vi "command stage.vi"(9 "Error In":errorcluster, 11 "Command Stage":T1={"dx (um) (0 -> ignore)"=0.0, "dy (um) (0 -> ignore)"=0.0, "dz (um) (0 -> ignore)"=0.0, "Re-center x,y"=FALSE, "Re-center z"=FALSE, "x (um) (-1 -> ignore)"=-1.0, "y (um) (-1 -> ignore)"=-1.0, "z (um) (-1 -> ignore)"=-1.0}) -> (1 "Error Out":errorcluster)   [LabVIEW 2014]
uses:
  Stage Control/Stage SubVis/move stage.ctl
  Stage Control/Stage SubVis/user event out globals - SubVI.vi
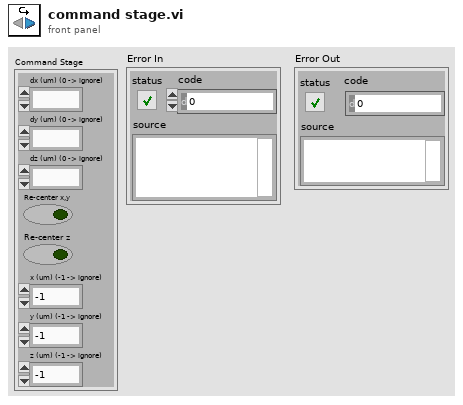
[diagram p1: front panel]
types:
  T1 = typedef "move stage.ctl" = cluster{"dx (um) (0 -> ignore)":ext, "dy (um) (0 -> ignore)":ext, "dz (um) (0 -> ignore)":ext, "Re-center x,y":bool, "Re-center z":bool, "x (um) (-1 -> ignore)":dbl, "y (um) (-1 -> ignore)":dbl, "z (um) (-1 -> ignore)":dbl}
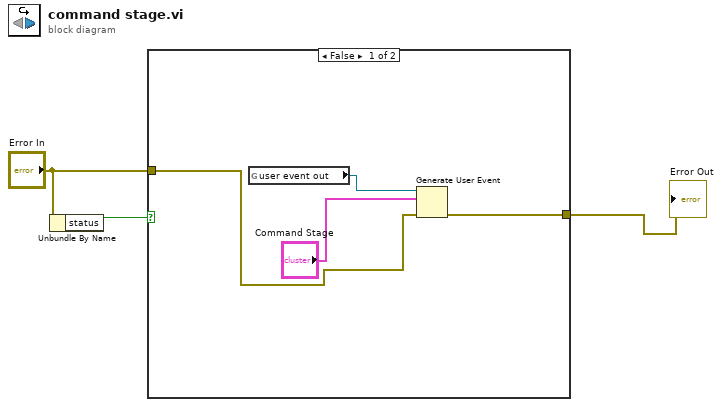
[diagram p0: block diagram]
diagram:
  n1 = Unbundle By Name("Error In") -> ("status"=w3:bool)
  n2 = case shown="False" w3 {
    tunnel: "Error In" -> [w5 w8]
    tunnel: [w4 w8] -> w1
    frame False {
      n3 = global read "user event out globals - SubVI.vi" "user event out"() -> (w7:refnum<user-event>)
      n4 = Generate User Event(user event=w7, event data cluster="Command Stage", error in=w5) -> (error out=w4:errorcluster)  [unwired: 1 in, 1 out]
    }
    frame True {
    }
  }
  "Error Out" <- w1
